vi "Current date.vi"() -> ()   [LabVIEW 2017]
panel:
  out "CAPACITY":dbl
  out "ACTUAL TIME":dbl
  out "BD RUNNING STATUS":bool
  in  "escalation number":string
  out "escalation PHN NO IND":bool
  out "PHONE NUMBER IND":bool
  in  "PHONE NUMBER":string
  in  "Current Date":string
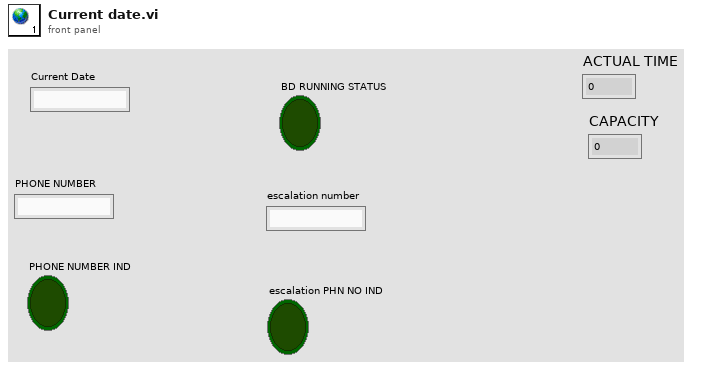
[diagram p1: front panel]
diagram:
